vi "power_correction.vi"(9 "Air humidity":dbl, 10 "Air temp":dbl, 11 "Ambient air press.":dbl) -> (2 "Numeric":dbl, 3 "Numeric 2":dbl)   [LabVIEW 2014]
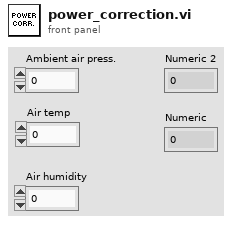
[diagram p1: front panel]
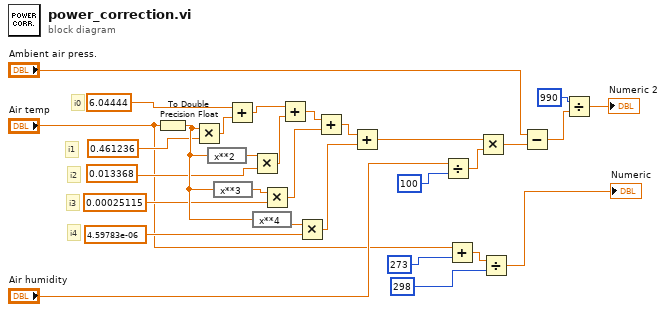
[diagram p0: block diagram]
diagram:
  # "i4"
  # "i3"
  # "i2"
  # "i1"
  # "i0"
  n1 = To Double Precision Float(number="Air temp") -> (double precision float=w28:dbl)
  n2 = Multiply(x=w28, y=0.461236) -> (x*y=w17:dbl)
  n3 = expression code="x**2"(w28) -> (w15:dbl)
  n4 = expression code="x**3"(w28) -> (w11:dbl)
  n5 = Add(x=6.04444, y=w17) -> (x+y=w16:dbl)
  n6 = Multiply(x=w15, y=0.013368) -> (x*y=w13:dbl)
  n7 = expression code="x**4"(w28) -> (w7:dbl)
  n8 = Multiply(x=w11, y=0.00025115) -> (x*y=w10:dbl)
  n9 = Add(x=w16, y=w13) -> (x+y=w9:dbl)
  n10 = Multiply(x=w7, y=4.59783e-06) -> (x*y=w6:dbl)
  n11 = Add(x=w9, y=w10) -> (x+y=w26:dbl)
  n12 = Add(x=w26, y=w6) -> (x+y=w4:dbl)
  n13 = Divide(x="Air humidity", y=100) -> (x/y=w3:dbl)
  n14 = Add(x="Air temp", y=273) -> (x+y=w22:dbl)
  n15 = Multiply(x=w4, y=w3) -> (x*y=w27:dbl)
  n16 = Divide(x=w22, y=298) -> (x/y=→"Numeric":dbl)
  n17 = Subtract(x="Ambient air press.", y=w27) -> (x-y=w2:dbl)
  n18 = Divide(x=990, y=w2) -> (x/y=→"Numeric 2":dbl)
